vi "Crash Test Dummy.vi"() -> ()   [LabVIEW 2014]
uses:
  <vilib>/MakerHub/LINX/Private/Utilties/Target Management/Install LV Data.ctl
  C:/Program Files (x86)/National Instruments/LabVIEW 2014/vi.lib/MakerHub/LINX/Resources/Renci.SshNet.dll
  Resources/Renci.SshNet.dll
  <vilib>/MakerHub/LINX/Private/Utilties/Target Management/Target Info.ctl
  <vilib>/MakerHub/LINX/LMH-LINX.lvlib
panel:
  out "Install LV Data in":T1={"SSH Session"=refnum, "Status Log"="", "Detailed Log"="", "Credentials"={"Hostname or IP"="192.168.7.2", "Username"="root", "Password"=""}, "Target Info"={"OS Version"="", "CPU"="", "Systemd Version"="", "Internet Access"=FALSE, "Device Type"=""}}
  out "Numeric Control":i32
  out "Error Out":errorcluster
  out "Connected?":bool
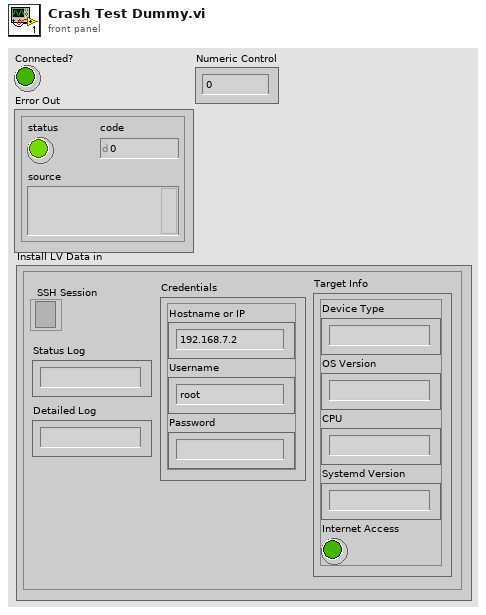
[diagram p1: front panel]
types:
  T1 = typedef "LMH-LINX.lvlib/Install LV Data.ctl" = cluster{"SSH Session":refnum<k24>, "Status Log":string, "Detailed Log":string, "Credentials":cluster{"Hostname or IP":string, "Username":string, "Password":string}, "Target Info":T2}
  T2 = typedef "LMH-LINX.lvlib/Target Info.ctl" = cluster{"OS Version":string, "CPU":string, "Systemd Version":string, "Internet Access":bool, "Device Type":string}
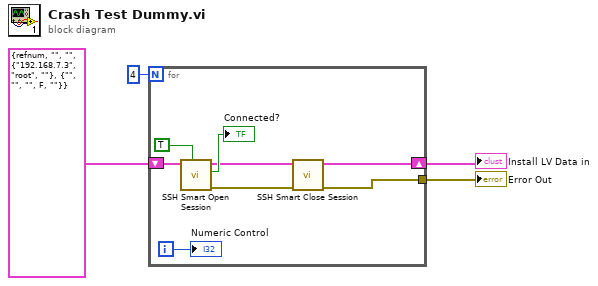
[diagram p0: block diagram]
diagram:
  n1 = for {
    N: 4 -> [_]
    tunnel: [w8] -> w3
    shift-right: [w5] -> w1
    shift-left: T1 {"SSH Session"=refnum, "Status Log"="", "Detailed Log"="", "Credentials"={"Hostname or IP"="192.168.7.3", "Username"="root", "Password"=""}, "Target Info"={"OS Version"="", "CPU"="", "Systemd Version"="", "Internet Access"=FALSE, "Device Type"=""}} ("Install LV Data in") -> [w12]
    i -> [w7]
    n2 = call <vilib>:"SSH Smart Open Session.vi"("Force Reconnect?"=TRUE, "Install LV Data in"=w12) -> ("Error Out"=w9:errorcluster, "Connected?"=→"Connected?":bool, "Install LV Data out"=w6:T1)  [unwired: 6 in, 1 out]
    n3 = call <vilib>:"SSH Smart Close Session.vi"("Error In"=w9, "Install LV Data"=w6) -> ("Error Out"=w8:errorcluster, "Install LV Data"=w5:T1)  [unwired: 8 in]
    "Numeric Control" <- w7
  }
  "Error Out" <- w3
  "Install LV Data in" <- w1
